vi "ReportGenerator.vi"() -> ()   [LabVIEW 2016]
uses:
  <vilib>/Utility/file.llb/Read Delimited Spreadsheet (string).vi
panel:
  in  "Output Text file(.txt)":path
  in  "Number of Students":i32
  in  "Input Excel file(.csv)":path
  # "REPORT GENERATOR"
  # "User Guide:\n\n      1.  Select the excelsheet (.csv format) which is to be manipulated.\n      2.  Select the text file (.txt format) where the report should be generated.\n      3. Select the number of students in the list to generate the report for.\n      4. Execute the program."
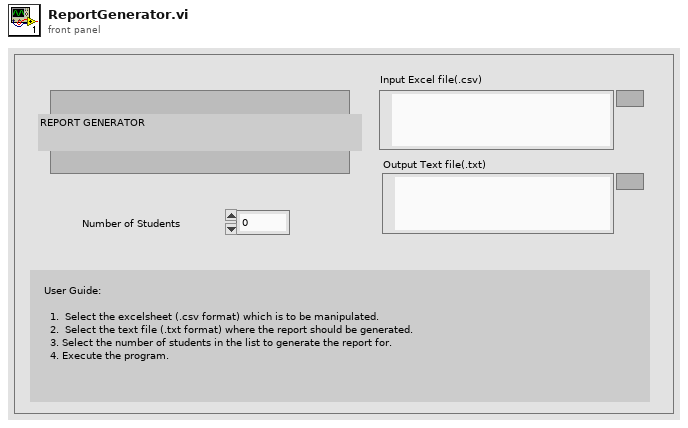
[diagram p1: front panel]
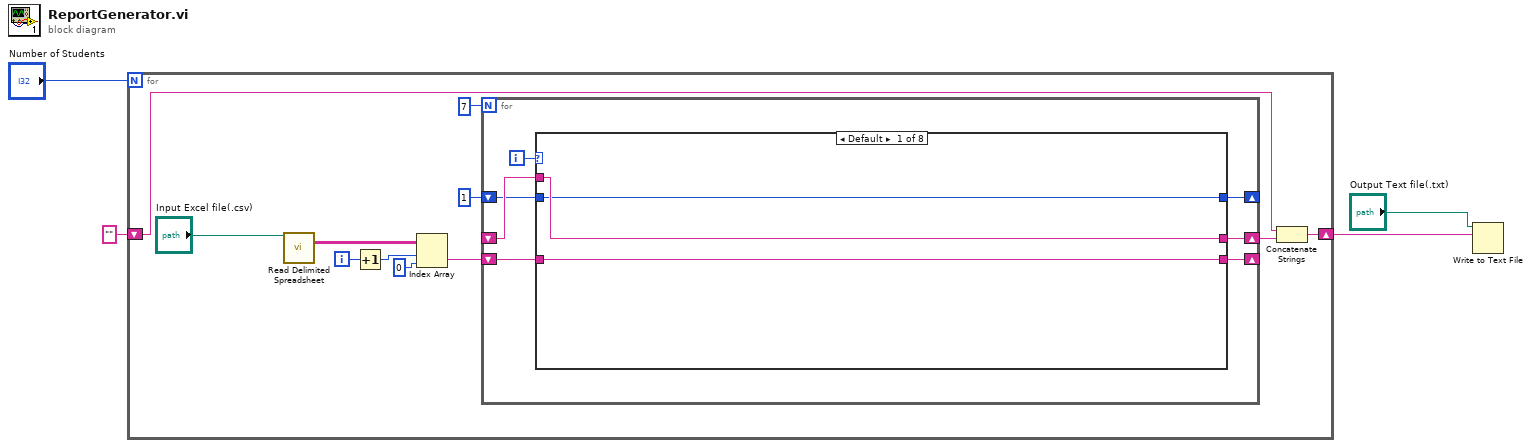
[diagram p0: block diagram]
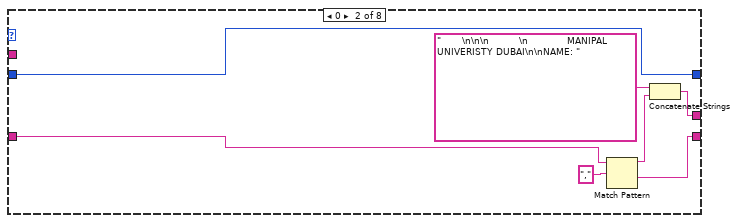
[diagram p2: hidden frame]
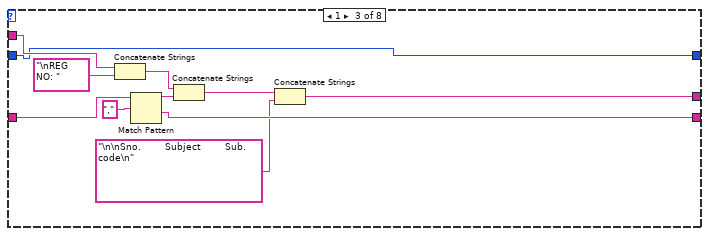
[diagram p3: hidden frame]
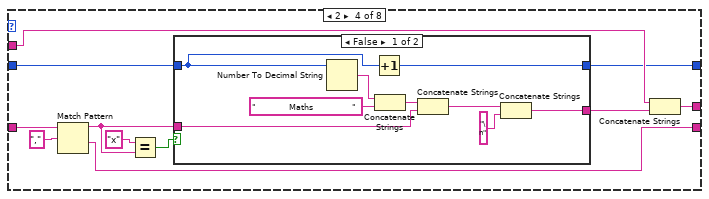
[diagram p4: hidden frame]
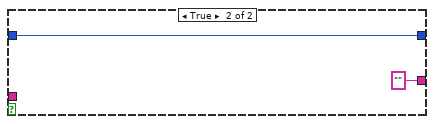
[diagram p5: hidden frame]
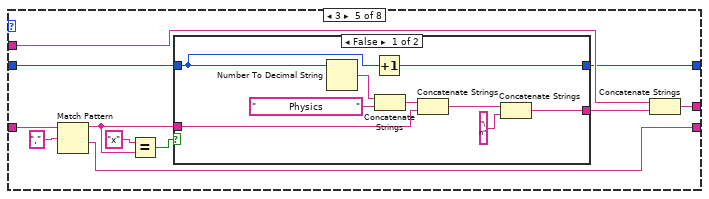
[diagram p6: hidden frame]
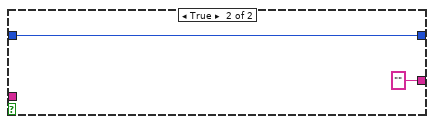
[diagram p7: hidden frame]
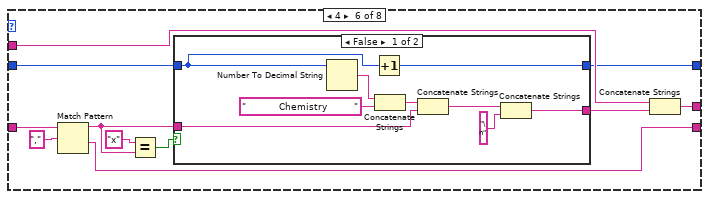
[diagram p8: hidden frame]
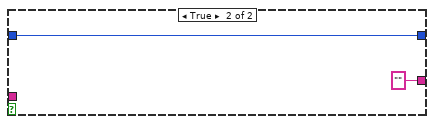
[diagram p9: hidden frame]
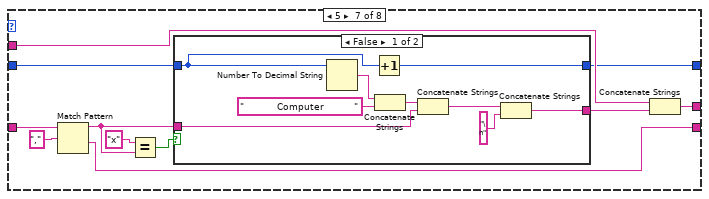
[diagram p10: hidden frame]
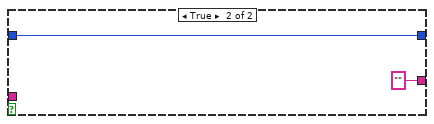
[diagram p11: hidden frame]
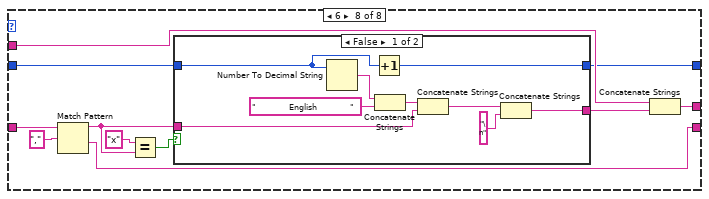
[diagram p12: hidden frame]
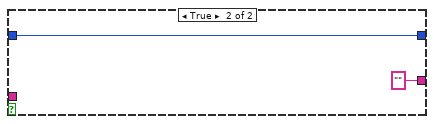
[diagram p13: hidden frame]
diagram:
  n1 = for {
    N: "Number of Students" -> [_]
    shift-right: [w7] -> w2
    shift-left: "" -> [w5]
    i -> [w9]
    n2 = call-poly <vilib>:"Read Delimited Spreadsheet.vi"("file path (dialog if empty)"="Input Excel file(.csv)") -> ("all rows"=w10:string[][])  [unwired: 9 in, 5 out]
    n3 = Increment(x=w9) -> (x+1=w8:i32)
    n4 = Index Array(array=w10, index (row)=w8, index (col)=0 ("disabled index (col)")) -> (element=w13:string)
    n5 = for {
      N: 7 -> [_]
      shift-right: [w20] -> _
      shift-left: w13 -> [w21]
      shift-right: [w19] -> w6
      shift-left: _ -> [w18]
      shift-right: [w16] -> _
      shift-left: 1 -> [w17]
      i -> [w22]
      n6 = case shown="Default" w22 {
        tunnel: w21 -> [w23 w32 w43 w53 w75 w97 w119 w141]
        tunnel: [w23 w30 w41 w51 w73 w95 w117 w139] -> w20
        tunnel: [w25 w27 w35 w46 w68 w90 w112 w134] -> w19
        tunnel: w18 -> [w25 _ w40 w54 w76 w98 w120 w142]
        tunnel: w17 -> [w24 w26 w33 w45 w67 w89 w111 w133]
        tunnel: [w24 w26 w33 w44 w66 w88 w110 w132] -> w16
        frame Default {
        }
        frame 0 {
          n7 = Match Pattern(string=w32, regular expression=",") -> (before substring=w29:string, after substring=w30:string)  [unwired: 1 in, 2 out]
          n8 = Concatenate Strings("       \n\n\n          \n             MANIPAL UNIVERISTY DUBAI\n\nNAME: " ("string"), w29) -> (w27:string)
        }
        frame 1 {
          n9 = Concatenate Strings(w40, "\nREG NO: " ("string")) -> (w38:string)
          n10 = Match Pattern(string=w43, regular expression=",") -> (before substring=w37:string, after substring=w41:string)  [unwired: 1 in, 2 out]
          n11 = Concatenate Strings(w38, w37) -> (w36:string)
          n12 = Concatenate Strings(w36, "\n\nSno.        Subject        Sub.code\n" ("string")) -> (w35:string)
        }
        frame 2 {
          n13 = Match Pattern(string=w53, regular expression=",") -> (before substring=w48:string, after substring=w51:string)  [unwired: 1 in, 2 out]
          n14 = Equal?(x="x", y=w48) -> (x = y?=w49:bool)
          n15 = case shown="False" w49 {
            tunnel: w48 -> [w58 _]
            tunnel: [w55 ""] -> w47
            tunnel: w45 -> [w62 w65]
            tunnel: [w61 w65] -> w44
            frame False {
              n16 = Number To Decimal String(number=w62) -> (decimal integer string=w63:string)  [unwired: 1 in]
              n17 = Increment(x=w62) -> (x+1=w61:i32)
              n18 = Concatenate Strings(w63, "           Maths             " ("string")) -> (w59:string)
              n19 = Concatenate Strings(w59, w58) -> (w57:string)
              n20 = Concatenate Strings(w57, "\n" ("string")) -> (w55:string)
            }
            frame True {
            }
          }
          n21 = Concatenate Strings(w54, w47) -> (w46:string)
        }
        frame 3 {
          n22 = Match Pattern(string=w75, regular expression=",") -> (before substring=w70:string, after substring=w73:string)  [unwired: 1 in, 2 out]
          n23 = Equal?(x="x", y=w70) -> (x = y?=w71:bool)
          n24 = case shown="False" w71 {
            tunnel: w70 -> [w80 _]
            tunnel: [w77 ""] -> w69
            tunnel: w67 -> [w84 w87]
            tunnel: [w83 w87] -> w66
            frame False {
              n25 = Number To Decimal String(number=w84) -> (decimal integer string=w85:string)  [unwired: 1 in]
              n26 = Increment(x=w84) -> (x+1=w83:i32)
              n27 = Concatenate Strings(w85, "           Physics           " ("string")) -> (w81:string)
              n28 = Concatenate Strings(w81, w80) -> (w79:string)
              n29 = Concatenate Strings(w79, "\n" ("string")) -> (w77:string)
            }
            frame True {
            }
          }
          n30 = Concatenate Strings(w76, w69) -> (w68:string)
        }
        frame 4 {
          n31 = Match Pattern(string=w97, regular expression=",") -> (before substring=w92:string, after substring=w95:string)  [unwired: 1 in, 2 out]
          n32 = Equal?(x="x", y=w92) -> (x = y?=w93:bool)
          n33 = case shown="False" w93 {
            tunnel: w92 -> [w102 _]
            tunnel: [w99 ""] -> w91
            tunnel: w89 -> [w106 w109]
            tunnel: [w105 w109] -> w88
            frame False {
              n34 = Number To Decimal String(number=w106) -> (decimal integer string=w107:string)  [unwired: 1 in]
              n35 = Increment(x=w106) -> (x+1=w105:i32)
              n36 = Concatenate Strings(w107, "           Chemistry         " ("string")) -> (w103:string)
              n37 = Concatenate Strings(w103, w102) -> (w101:string)
              n38 = Concatenate Strings(w101, "\n" ("string")) -> (w99:string)
            }
            frame True {
            }
          }
          n39 = Concatenate Strings(w98, w91) -> (w90:string)
        }
        frame 5 {
          n40 = Match Pattern(string=w119, regular expression=",") -> (before substring=w114:string, after substring=w117:string)  [unwired: 1 in, 2 out]
          n41 = Equal?(x="x", y=w114) -> (x = y?=w115:bool)
          n42 = case shown="False" w115 {
            tunnel: w114 -> [w124 _]
            tunnel: [w121 ""] -> w113
            tunnel: w111 -> [w128 w131]
            tunnel: [w127 w131] -> w110
            frame False {
              n43 = Number To Decimal String(number=w128) -> (decimal integer string=w129:string)  [unwired: 1 in]
              n44 = Increment(x=w128) -> (x+1=w127:i32)
              n45 = Concatenate Strings(w129, "           Computer          " ("string")) -> (w125:string)
              n46 = Concatenate Strings(w125, w124) -> (w123:string)
              n47 = Concatenate Strings(w123, "\n" ("string")) -> (w121:string)
            }
            frame True {
            }
          }
          n48 = Concatenate Strings(w120, w113) -> (w112:string)
        }
        frame 6 {
          n49 = Match Pattern(string=w141, regular expression=",") -> (before substring=w136:string, after substring=w139:string)  [unwired: 1 in, 2 out]
          n50 = Equal?(x="x", y=w136) -> (x = y?=w137:bool)
          n51 = case shown="False" w137 {
            tunnel: w136 -> [w146 _]
            tunnel: [w143 ""] -> w135
            tunnel: w133 -> [w150 w153]
            tunnel: [w149 w153] -> w132
            frame False {
              n52 = Number To Decimal String(number=w150) -> (decimal integer string=w151:string)  [unwired: 1 in]
              n53 = Increment(x=w150) -> (x+1=w149:i32)
              n54 = Concatenate Strings(w151, "           English           " ("string")) -> (w147:string)
              n55 = Concatenate Strings(w147, w146) -> (w145:string)
              n56 = Concatenate Strings(w145, "\n" ("string")) -> (w143:string)
            }
            frame True {
            }
          }
          n57 = Concatenate Strings(w142, w135) -> (w134:string)
        }
      }
    }
    n58 = Concatenate Strings(w5, w6) -> (w7:string)
  }
  n59 = Write to Text File(file (use dialog)="Output Text file(.txt)", text=w2) -> ()  [unwired: 2 in, 3 out]
